vi "Configure Trigger (Timeout).vi"(0 "VISA resource name":refnum<visa-resource-name>, 5 "Source (1: Channel 1)":i32(ring)=1 items=["Channel 1"=1, "Channel 2"=2, "Channel 3"=3, "Channel 4"=4], 9 "Edge Type (0: Positive)":i32(ring) items=["Positive", "Negative", "Either"], 11 "error in (no error)":errorcluster, 12 "Timeout (1E-6 s)":dbl=1e-06, 13 "Trigger Level (0)":dbl) -> (4 "VISA resource name out":refnum<visa-resource-name>, 15 "error out":errorcluster)   [LabVIEW 2015, in "ZhiYuan ZDS Series for TCP.lvlib"]
doc: "Configures the setting for timeout trigger.\n\nNote: This VI is only applicable for DS 2000 Series."
uses:
  ZhiYuan ZDS Series for TCP.lvlib
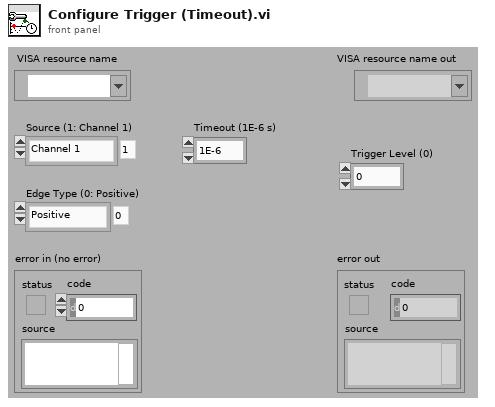
[diagram p1: front panel]
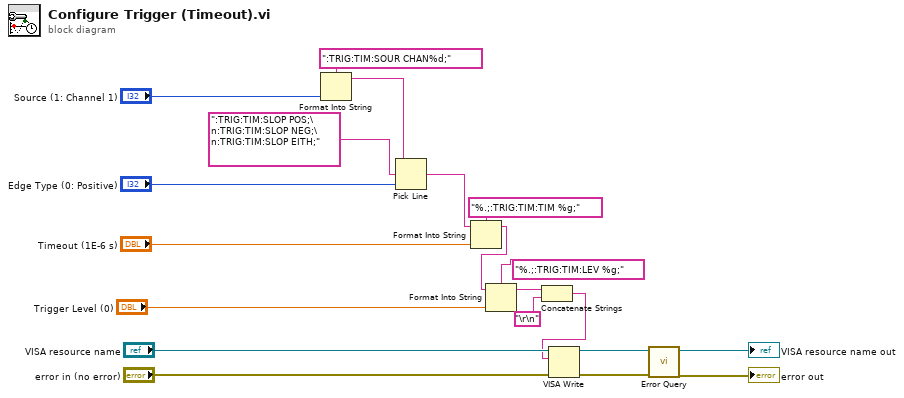
[diagram p0: block diagram]
diagram:
  n1 = Format Into String(format string=":TRIG:TIM:SOUR CHAN%d;", "Source (1: Channel 1)") -> (resulting string=w16:string)  [unwired: 2 in, 1 out]
  n2 = Pick Line(string ("")=w16, multi-line string=":TRIG:TIM:SLOP POS;\n:TRIG:TIM:SLOP NEG;\n:TRIG:TIM:SLOP EITH;", line index="Edge Type (0: Positive)") -> (output string=w15:string)
  n3 = Format Into String(format string="%.;:TRIG:TIM:TIM %g;", initial string=w15, "Timeout (1E-6 s)") -> (resulting string=w6:string)  [unwired: 1 in, 1 out]
  n4 = Format Into String(format string="%.;:TRIG:TIM:LEV %g;", initial string=w6, "Trigger Level (0)") -> (resulting string=w3:string)  [unwired: 1 in, 1 out]
  n5 = Concatenate Strings(w3, "\r\n") -> (w1:string)
  n6 = VISA Write(VISA resource name="VISA resource name", write buffer=w1, error in (no error)="error in (no error)") -> (VISA resource name out=w10:refnum<visa-resource-name>, error out=w9:errorcluster)  [unwired: 1 out]
  n7 = call "Error Query.vi"("error in (no error)"=w9, "VISA resource name"=w10) -> ("error out"=→"error out":errorcluster, "VISA resource name out"=→"VISA resource name out":refnum<visa-resource-name>)  [unwired: 6 in, 2 out]
